vi "Fast_response_stats.vi"(0 "U":dbl[](array[numeric]) format="%.2f", 1 "Index":i32, 11 "Shift in":dbl[](array[numeric]) format="%.2f", 12 "Block No":i32=1) -> (4 "Results file string array":string[](array[string]), 15 "Shift out":dbl[](array[numeric]) format="%.2f")   [LabVIEW 2010]
uses:
  Globals/Meas_global.vi
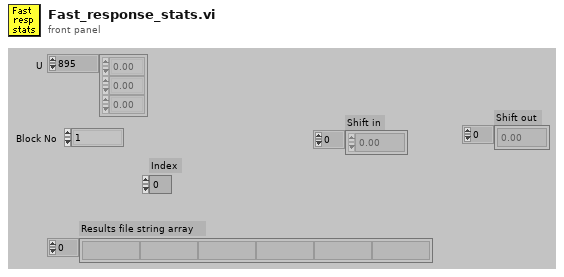
[diagram p1: front panel]
types:
  T1 = typedef "Velocity_cluster.ctl" = cluster{"Name":string, "U":dbl, "u^2":dbl, "u^3/(u^2)^(1.5)":dbl, "u^4/(u^2)^2 -3":dbl, "% u'/U":dbl, "Mean % Err":dbl, "u^4":dbl}
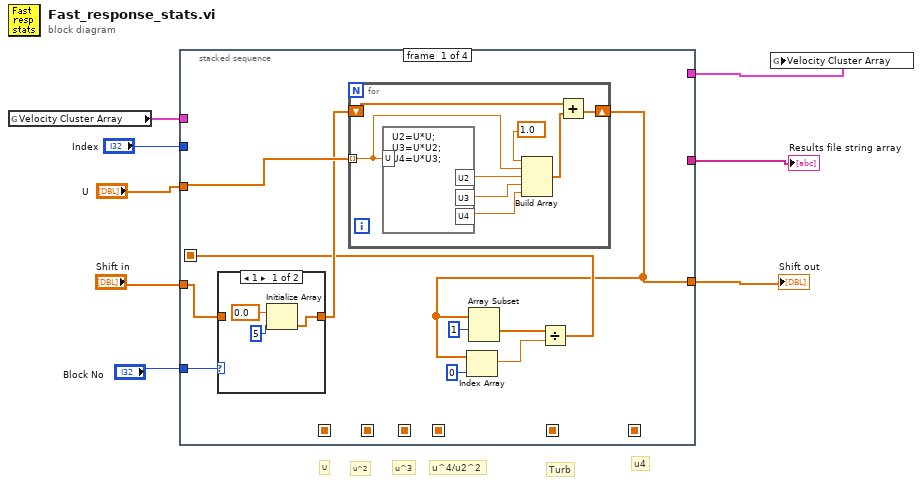
[diagram p0: block diagram]
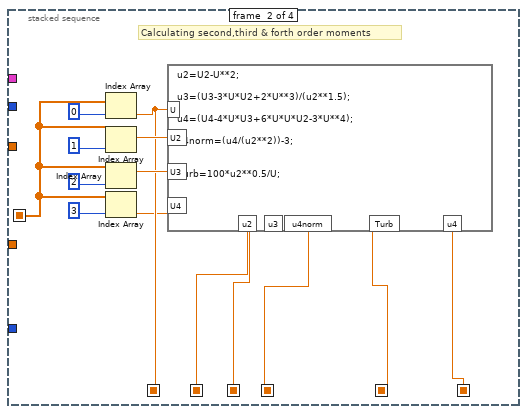
[diagram p3: hidden frame]
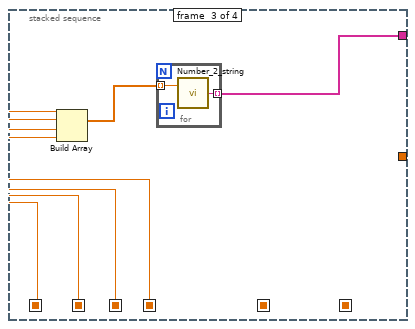
[diagram p4: hidden frame]
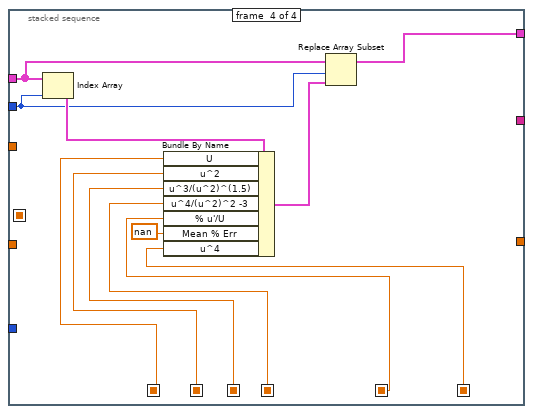
[diagram p5: hidden frame]
diagram:
  # "u4"
  # "u^4/u2^2"
  # "u^3"
  # "Turb"
  # "U"
  # "u^2"
  n1 = global read "Meas_global.vi" "Velocity Cluster Array"() -> (w5:T1[])
  n2 = stacked-sequence {
    seq-local: [_ w41 _ _] -> [_ _ w49 w58]
    seq-local: [w10 _ _ _] -> [_ w34 _ _]
    seq-local: [_ w33 _ _] -> [_ _ w50 w59]
    seq-local: [_ w42 _ _] -> [_ _ _ w57]
    seq-local: [_ w36 _ _] -> [_ _ w48 w56]
    seq-local: [_ w35 _ _] -> [_ _ w47 w55]
    seq-local: [_ w31 _ _] -> [_ _ _ w53]
    tunnel: "U" -> [w18 _ _ _]
    tunnel: [w9 _ _ _] -> w7
    tunnel: "Shift in" -> [w12 _ _ _]
    tunnel: [_ _ w45 _] -> w6
    tunnel: w5 -> [_ _ _ w62]
    tunnel: "Index" -> [_ _ _ w61]
    tunnel: [_ _ _ w60] -> w3
    tunnel: "Block No" -> [w13 _ _ _]
    frame #0 {
      n3 = case shown="1" w13 {
        tunnel: [w19 w22] -> w11
        tunnel: w12 -> [_ w22]
        frame 1 {
          n4 = Initialize Array(0.0 ("Element Data"), 5 ("Dimension Size")) -> (w19:dbl[])
        }
        frame 2, Default {
        }
      }
      n5 = for {
        shift-right: [w29] -> w9
        shift-left: w11 -> [w30]
        tunnel: w18 -> [w23] mode=indexing
        n6 = formula code="U2=U*U;\nU3=U*U2;\nU4=U*U3;"("U"=w23) -> ("U2"=w27:dbl, "U3"=w26:dbl, "U4"=w25:dbl)
        n7 = Build Array(1.0 ("Input Element"), w23, w27, w26, w25) -> (w28:dbl[])
        n8 = Add(x=w30, y=w28) -> (x+y=w29:dbl[])
      }
      n9 = Index Array(array=w9, index=0 ("Index")) -> (element=w14:dbl)
      n10 = Array Subset(array=w9, index=1 ("Array Index")) -> (w15:dbl[])  [unwired: 1 in]
      n11 = Divide(x=w15, y=w14) -> (x/y=w10:dbl[])
    }
    frame #1 {
      # "Calculating second,third & forth order moments"
      n12 = Index Array(array=w34, index=0) -> (element=w33:dbl)
      n13 = Index Array(array=w34, index=1) -> (element=w38:dbl)
      n14 = Index Array(array=w34, index=2) -> (element=w37:dbl)
      n15 = Index Array(array=w34, index=3) -> (element=w32:dbl)
      n16 = formula code="u2=U2-U**2;\n\nu3=(U3-3*U*U2+2*U**3)/(u2**1.5);\n\nu4=(U4-4*U*U3+6*U*U*U2-3*U**4);\n\nu4norm=(u4/(u2**2))-3;\n\n\nTurb=100*u2**0.5/U;"("U"=w33, "U2"=w38, "U3"=w37, "U4"=w32) -> ("u2"=w41:dbl, "Turb"=w42:dbl, "u3"=w36:dbl, "u4norm"=w35:dbl, "u4"=w31:dbl)
    }
    frame #2 {
      n17 = Build Array(w50, w49, w48, w47) -> (w46:dbl[])
      n18 = for {
        tunnel: w46 -> [w52] mode=indexing
        tunnel: [w51] -> w45 mode=indexing
        n19 = call "Number_2_string.vi"("number"=w52) -> ("String"=w51:string)  [unwired: 1 in]
      }
    }
    frame #3 {
      n20 = Index Array(array=w62, index=w61) -> (element=w64:T1)
      n21 = Bundle By Name(cluster=w64, "U"=w59, "u^2"=w58, "u^3/(u^2)^(1.5)"=w56, "u^4/(u^2)^2 -3"=w55, "% u'/U"=w57, "Mean % Err"=nan ("u^3/(u^2)^(1.5)"), "u^4"=w53) -> (w63:T1)
      n22 = Replace Array Subset(array=w62, new element=w63, index=w61) -> (w60:T1[])
    }
  }
  "Shift out" <- w7
  "Results file string array" <- w6
  n23 = global write "Meas_global.vi" "Velocity Cluster Array"(w3) -> ()
